vi "Write U8 External Payload.vi"(8 "error in (no error)":errorcluster, 9 "Timeout (ms)":i32, 10 "U8 With Header in":u8[](array[numeric]), 11 "CIFFIFO in":refnum<class "CIF_CIPC_Fifo_U8.lvclass">) -> (0 "error out":errorcluster, 1 "timed out?":bool, 2 "U8 With Header out":u8[](array[numeric]), 3 "CIFFIFO out":refnum<class "CIF_CIPC_Fifo_U8.lvclass">)   [LabVIEW 2021, in "CIF_CIPC_Fifo_U8.lvclass"]
doc: "Write the full payload bytes, including the encoded header. This is intended for advanced applications where the full buffer was received externally. The header will still be updated with the new T_TX"
uses:
  CIF_CIPC_Fifo_U8.lvclass
  D:/dev/Packages/CIF_Channels_Core/src/CIPC_Channels/CIF_CIPC_Chan/CIF_CIPC_Chn.lvclass
  D:/dev/Packages/CIF_Channels_Core/src/CIFChannels/CIFChannels.lvclass
  CIFChannels/CIFChannels.lvclass/CIFChannels.ctl
  CIF_CIPC_Chan/CIF_CIPC_Chn.lvclass/CIF_CIPC_Chn.ctl
  ChannelCommon/typedef/TimeStamps.ctl
  <vilib>/CIF Foundation/CIF Utilities/Statistics/I64/Stats_I64_CIF_U.lvclass/Stats_I64_CIF_U.ctl
  CIF_CIPC_Chan/Accessors/Read Buffer Configuration.vi
  CIF_CIPC_Chan/SubVIs/Check Writer Backpressure.vi/7796537b-0e69-421b-96bb-30a861203fb6.vi
  CIFChannels/Accessors/Read FIFO Backpressure.vi
  <vilib>/CIF Foundation/CIF Utilities/DataTypes/Flatten Unflatten/Unflatten U64.vi
  <vilib>/CIF Foundation/CIF Utilities/DataTypes/Flatten Unflatten/Unflatten I64.vi
  ChannelCommon/Utilities/Add Error.vi
  CIFChannels/Utilities/Update Channel Benchmark.vi
  SubVIs/Core Write U8 FIFO.vi/1bad10da-a98b-49ee-b03a-18b497e396df.vi
  SubVIs/Core Write U8 FIFO.vi/70f860b1-5d4a-43dc-b0c2-c9446e8447f7.vi
  CIF_CIPC_Chan/Accessors/Read CIPC Channel.vi
  SubVIs/Core Write U8 FIFO.vi/40f8d1bb-2a62-444a-8ee6-d4d6c496dc12.vi
  CIFChannels/Accessors/Read FIFO Header.vi
  CIF_CIPC_Chan/SubVIs/Check Writer Backpressure.vi/7796537b-0e69-421b-96bb-30a861203fb6.vi/a816fde8-6378-45f6-992d-c1f6c5777b8d.vi
  <vilib>/CIF Foundation/CIF CIPC/SubVIs/Get Element Write Position.vi
  <vilib>/CIF Foundation/CIF CIPC/Utilities/Get Size.vi
  <vilib>/CIF Foundation/CIF Utilities/Statistics/I64/X1 minus X0.vi
  <vilib>/CIF Foundation/CIF Utilities/Time/System Time/Get System Time.vi
  <vilib>/CIF Foundation/CIF CIPC/SubVIs/Check Error.vi
  <vilib>/CIF Foundation/CIF CIPC/SubVIs/Notify Of New Write.vi
  <vilib>/CIF Foundation/CIF CIPC/SubVIs/Get dll Path.vi
  <vilib>/CIF Foundation/CIF CIPC/SubVIs/Wait For N Elements Available.vi
  <vilib>/CIF Foundation/CIF CIPC/SubVIs/Get Element Read Position.vi
  <vilib>/CIF Foundation/CIF CIPC/SubVIs/Set Element Read Position.vi
  <vilib>/CIF Foundation/CIF Utilities/Statistics/I64/X1 minus X0.vi/dfabcf33-0dbc-4041-80a5-3dc0c86d2989.vi
  <vilib>/CIF Foundation/CIF Utilities/Time/System Time/LabVIEW Time to TAI Time.vi
  <vilib>/CIF Foundation/CIF Utilities/Statistics/I64/X1 minus X0.vi/dfabcf33-0dbc-4041-80a5-3dc0c86d2989.vi/9eb60a9a-770f-4d2d-8b3f-8465c267ecc9.vi
  CIF_CIPC_Chan/CIF_CIPC_Chn.lvclass
  <vilib>/CIF Foundation/CIF CIPC/SubVIs/Check Error Core.vi
  <vilib>/CIF Foundation/CIF CIPC/SubVIs/Get Element Info Variant.vi
  <vilib>/CIF Foundation/CIF CIPC/SubVIs/Check Backpressure FIFO Space.vi
  ChannelCommon/Utilities/Add Error Core.vi
  CIF_CIPC_Fifo_U8.lvclass/CIF_CIPC_Fifo_U8.ctl
  CIFChannels/CIFChannels.lvclass
  ChannelCommon/ChannelCommon.lvlib
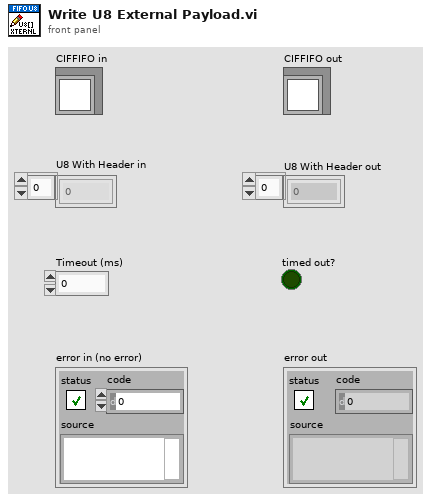
[diagram p1: front panel]
types:
  T1 = typedef "ChannelCommon.lvlib/TimeStamps.ctl" = cluster{"ClockID":u8, "T0":i64, "T_Out":i64}
  T2 = typedef "ChannelCommon.lvlib/FIFO Header.ctl" = cluster{"Length":u64, "T0":i64, "T_Out":i64, "T_Tx":i64, "Ctr":u64, "ClockID":u8}
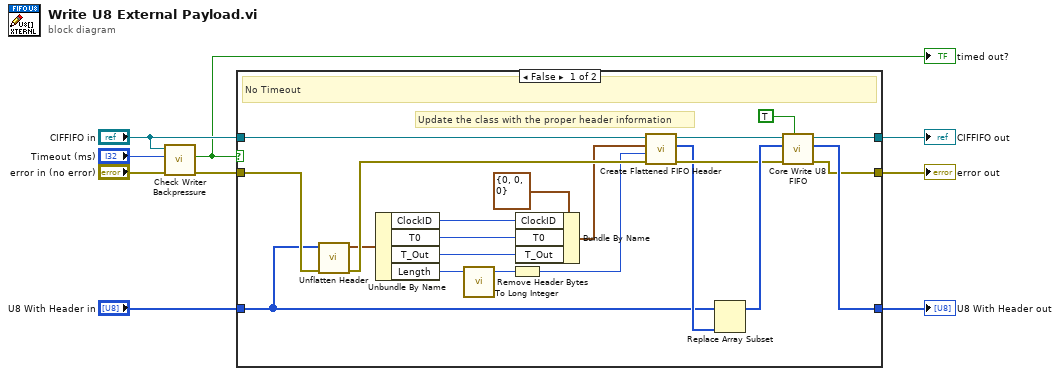
[diagram p0: block diagram]
diagram:
  n1 = call "Check Writer Backpressure.vi"("error in (no error)"="error in (no error)", "Timeout (ms)"="Timeout (ms)", "CIF_CIPC_Chn in"="CIFFIFO in") -> ("error out"=w9:errorcluster, "timed out?"=w5:bool)  [unwired: 7 in]
  "timed out?" <- w5
  n2 = case shown="False" w5 {
    tunnel: [w14 w33] -> w3
    tunnel: [w16 w32] -> w4
    tunnel: "CIFFIFO in" -> [w17 w32]
    tunnel: w9 -> [w13 w33]
    tunnel: [w15 w31] -> w2
    tunnel: "U8 With Header in" -> [w12 w31]
    frame False {
      # "Update the class with the proper header information"
      # "No Timeout"
      n3 = call "Unflatten Header.vi"("error in (no error)"=w13, "Flattened Data in"=w12) -> ("error out"=w26:errorcluster, "Header out"=w20:T2)  [unwired: 7 in, 1 out]
      n4 = Unbundle By Name(w20) -> ("ClockID"=w25:u8, "T0"=w24:i64, "T_Out"=w23:i64, "Length"=w11:u64)
      n5 = call "Remove Header Bytes.vi"("Bytes/Msg with header"=w11) -> ("Bytes/Msg without header"=w10:u64)  [unwired: 3 in]
      n6 = To Long Integer(number=w10) -> (32bit integer=w21:i32)
      n7 = Bundle By Name(cluster=T1 {"ClockID"=0, "T0"=0, "T_Out"=0} ("FIFO Timestamps"), "ClockID"=w25, "T0"=w24, "T_Out"=w23) -> (w22:T1)
      n8 = call "Create Flattened FIFO Header.vi"("error in (no error)"=w26, "Payload Length"=w21, "FIFO Timestamps"=w22, "CIFChannels in"=w17) -> ("error out"=w29:errorcluster, "Flattened FIFO Header"=w27:u8[], "CIFChannels out"=w28:refnum<class "CIF_CIPC_Fifo_U8.lvclass">)  [unwired: 5 in]
      n9 = Replace Array Subset(array=w12, new element=w27) -> (w30:u8[])  [unwired: 1 in]
      n10 = call "Core Write U8 FIFO.vi"("Includes Header"=TRUE, "error in (no error)"=w29, "U8 in"=w30, "CIFFIFO in"=w28) -> ("error out"=w14:errorcluster, "U8 out"=w15:u8[], "CIFFIFO out"=w16:refnum<class "CIF_CIPC_Fifo_U8.lvclass">)  [unwired: 5 in]
    }
    frame True {
      # "Timeout"
    }
  }
  "error out" <- w3
  "U8 With Header out" <- w2
  "CIFFIFO out" <- w4
